vi "AutoConfigureAdditionalMotionPlanes_19May2014.vi"(0 "Motion ROIs":T3(array[cluster]), 1 "Number of Motion Points":i32, 2 "Plane Params":T1={"XY Offset"=3, "Z Offset"=6, "Line Length"=12.0, "Box Size"=12.0, "Number of Planes Per Point"=3}, 5 "In Points":i32[][](array[numeric]), 7 "Grid Points":i32=10, 9 "Motion Rate (Hz)":dbl=10.0, 11 "error in (no error)":errorcluster, 12 "Scan Settings":T2, 13 "Scan Settings (um)":T2={"XStart"=-100, "XEnd"=100, "XNum"=250, "YStart"=-100, "YEnd"=100, "YNum"=250, "ZStart"=-50, "ZEnd"=50, "ZNum"=30}) -> (3 "X-Y Motion Points":i32[][](array[numeric]), 4 "Out Points":i32[][](array[numeric]), 6 "Total Motion Points":i32, 8 "Motion Increment":i32, 10 "Sampling Interval":dbl, 14 "Y-Z Motion Points":i32[][](array[numeric]), 15 "error out":errorcluster)   [LabVIEW 2012]
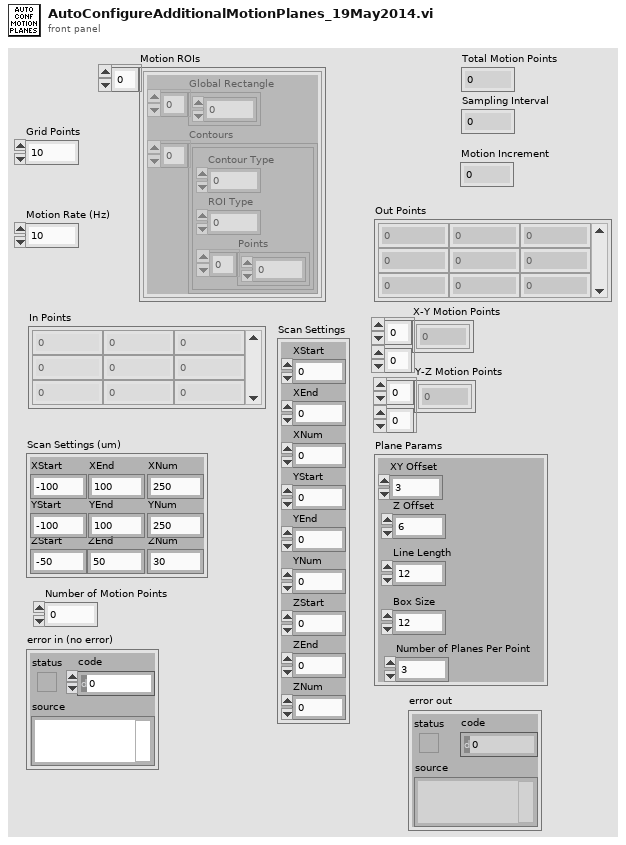
[diagram p1: front panel]
types:
  T1 = cluster{"XY Offset":i32, "Z Offset":i32, "Line Length":dbl, "Box Size":dbl, "Number of Planes Per Point":i32}
  T2 = cluster{"XStart":i32, "XEnd":i32, "XNum":i32, "YStart":i32, "YEnd":i32, "YNum":i32, "ZStart":i32, "ZEnd":i32, "ZNum":i32}
  T3 = cluster{"Global Rectangle":i32[], "Contours":cluster{"Contour Type":u32, "ROI Type":u32, "Points":i32[]}[]}[]
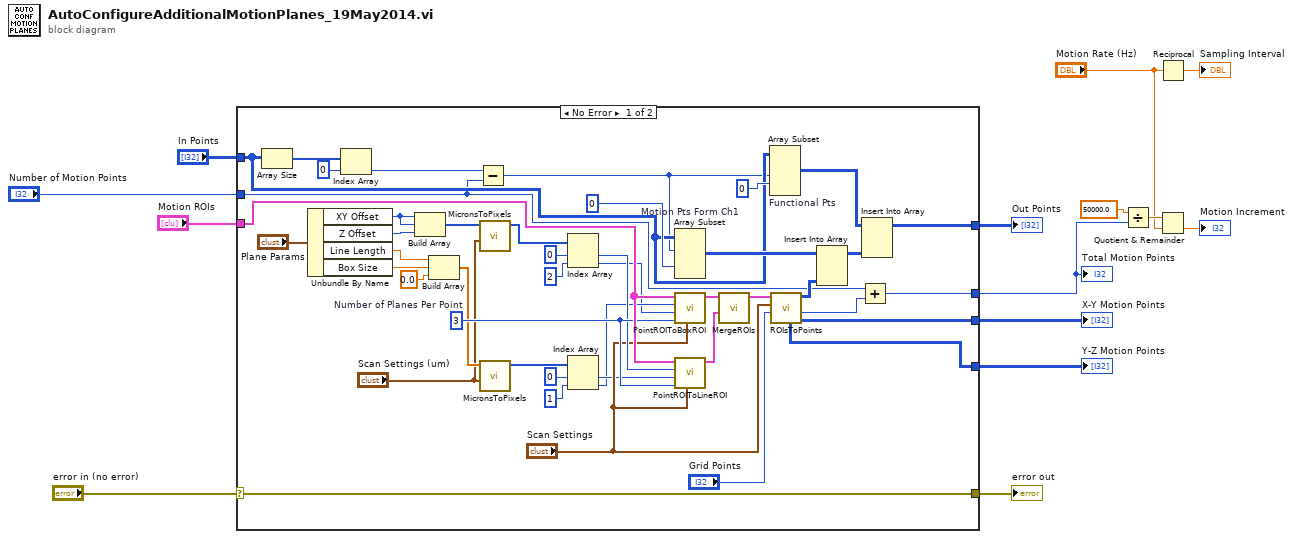
[diagram p0: block diagram]
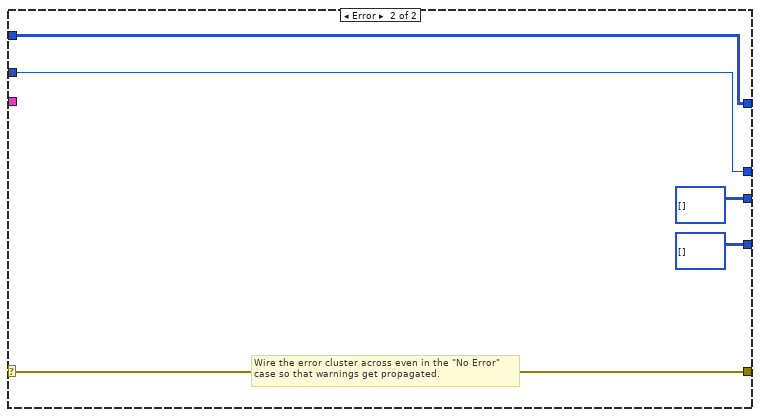
[diagram p2: hidden frame]
diagram:
  n1 = case shown="No Error" "error in (no error)" {
    selector: "error in (no error)" -> [w58 w63]
    tunnel: [w58 w63] -> w13
    tunnel: "Motion ROIs" -> [w57 _]
    tunnel: [w37 w62] -> w11
    tunnel: "In Points" -> [w36 w62]
    tunnel: [w34 w61] -> w7
    tunnel: "Number of Motion Points" -> [w33 w61]
    tunnel: [w31 i32[][] [] ("Y-Z Motion Points")] -> w2
    tunnel: [w30 i32[][] [] ("X-Y Motion Points")] -> w1
    frame No Error {
      w56 = 3  # Number of Planes Per Point
      n2 = Array Size(array=w36) -> (size(s)=w46:i32[])
      n3 = Unbundle By Name("Plane Params") -> ("XY Offset"=w27:i32, "Z Offset"=w26:i32, "Line Length"=w24:dbl, "Box Size"=w23:dbl)
      n4 = Index Array(array=w46, index=0) -> (element=w44:i32)
      n5 = Build Array(w27, w27, w26) -> (w28:i32[])
      n6 = Build Array(w24, w23, 0.0 ("element")) -> (w25:dbl[])
      n7 = Subtract(x=w44, y=w33) -> (x-y=w32:i32)
      n8 = call "MicronsToPixels.vi"("Scan Settings (um)"="Scan Settings (um)", "Microns (X,Y,Z)"=w28) -> ("Pixels (X,Y,Z)"=w53:i32[])  [unwired: 9 in]
      n9 = call "MicronsToPixels.vi"("Scan Settings (um)"="Scan Settings (um)", "Microns (X,Y,Z)"=w25) -> ("Pixels (X,Y,Z)"=w18:i32[])  [unwired: 9 in]
      n10 = Index Array(array=w53, index #1=0 ("index"), index #2=2 ("index")) -> (element #1=w50:i32, element #2=w15:i32)
      n11 = Index Array(array=w18, index #1=0 ("index"), index #2=1 ("index")) -> (element #1=w17:i32, element #2=w16:i32)
      n12 = Array Subset "Motion Pts Form Ch1"(array=w36, index (row)=w32, index (col)=0 ("index")) -> (w41:i32[][])  [unwired: 2 in]
      n13 = call "PointROIToBoxROI.vi"("Scan Settings"="Scan Settings", "Number of Boxes"=w56, "Box Offset Z (pixels)"=w15, "Box Size (pixels)"=w16, "PT ROIs"=w57) -> ("BOX ROIs"=w55:T3)  [unwired: 6 in]
      n14 = call "PointROIToLineROI.vi"("Scan Settings"="Scan Settings", "Number of Lines (Odd)"=w56, "Line Length (pixels)"=w17, "Line Offset X (pixels)"=w50, "PT ROIs"=w57) -> ("LINE ROIs"=w54:T3)  [unwired: 6 in]
      n15 = call "MergeROIs.vi"("ROI 2"=w54, "ROI 1"=w55) -> ("Merged ROI"=w49:T3)  [unwired: 9 in]
      n16 = Array Subset "Functional Pts"(array=w36, length (row)=w32, index (col)=0 ("index")) -> (w39:i32[][])  [unwired: 2 in]
      n17 = call "ROIsToPoints.vi"("GridPoints"="Grid Points", "Scan Settings"="Scan Settings", "ROI"=w49) -> ("X-Y Motion Points"=w30:i32[][], "Number of motion points"=w35:i32, "Points"=w40:i32[][], "Y-Z Motion Points"=w31:i32[][])  [unwired: 4 in, 1 out]
      n18 = Insert Into Array(array=w41, new element=w40) -> (w38:i32[][])  [unwired: 2 in]
      n19 = Add(x=w33, y=w35) -> (x+y=w34:i32)
      n20 = Insert Into Array(array=w39, new element=w38) -> (w37:i32[][])  [unwired: 2 in]
    }
    frame Error {
      # "Wire the error cluster across even in the \"No Error\"\ncase so that warnings get propagated."
    }
  }
  "error out" <- w13
  "Out Points" <- w11
  "Total Motion Points" <- w7
  "X-Y Motion Points" <- w1
  "Y-Z Motion Points" <- w2
  n21 = Divide(x=50000.0, y=w7) -> (x/y=w6:dbl)
  n22 = Reciprocal(x="Motion Rate (Hz)") -> (1/x=→"Sampling Interval":dbl)
  n23 = Quotient & Remainder(x=w6, y="Motion Rate (Hz)") -> (floor(x/y)=→"Motion Increment":dbl)  [unwired: 1 out]
